vi "DEMO.vi"() -> ()   [LabVIEW 2013, in "标准状态机模板.lvlib"]
uses:
  Control/Input Data.ctl
  Control/Output Data.ctl
panel:
  out "Output Data":T1
  in  "Input Data":T2
  in  "停止":bool
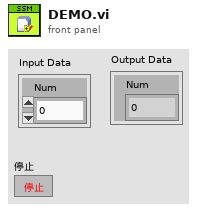
[diagram p1: front panel]
types:
  T1 = typedef "标准状态机模板.lvlib/Output Data.ctl" = cluster{"Num":dbl}
  T2 = typedef "标准状态机模板.lvlib/Input Data.ctl" = cluster{"Num":dbl}
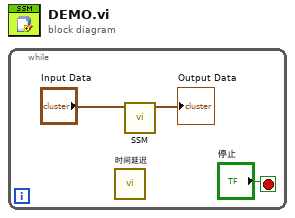
[diagram p0: block diagram]
diagram:
  n1 = while {
    stop <- "停止" stop-if-true
    n2 = call "时间延迟"() -> ()  [unwired: 11 in, 1 out]
    n3 = call "SSM.VI"("Input Data"="Input Data") -> ("Output Data"=→"Output Data":T1)  [unwired: 9 in, 1 out]
  }
